vi "DSF.Execution.Runtime.Plugin Manager.Load Classes.vi"(8 "error in (no error)":errorcluster, 10 "class paths":path[](array[path]), 11 "Plugin Manager in":refnum<class "DSF.Engine.Runtime.Plugin Manager.lvclass">) -> (0 "error out":errorcluster, 2 "objects":refnum<class>[](array[class]), 3 "Plugin Manager out":refnum<class "DSF.Engine.Runtime.Plugin Manager.lvclass">)   [LabVIEW 2016, in "DSF.Engine.lvlib" / "DSF.Engine.Runtime.Plugin Manager.lvclass"]
uses:
  DSF.Engine.Runtime.Plugin Manager.lvclass
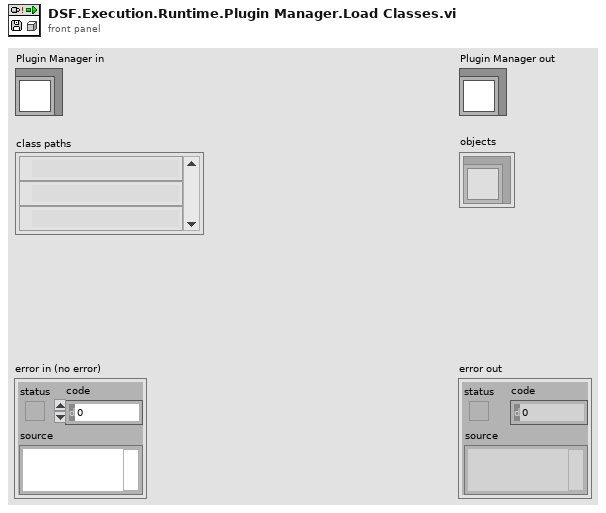
[diagram p1: front panel]
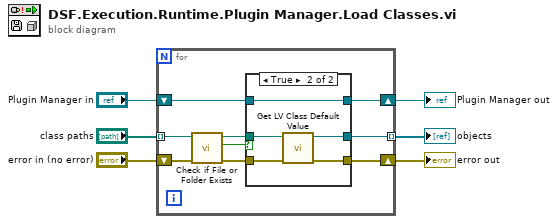
[diagram p0: block diagram]
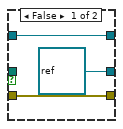
[diagram p2: hidden frame]
diagram:
  n1 = for {
    shift-right: [w10] -> w1
    shift-left: "error in (no error)" -> [w15]
    shift-right: [w7] -> w3
    shift-left: "Plugin Manager in" -> [w8]
    tunnel: "class paths" -> [w14] mode=indexing
    tunnel: [w9] -> w2 mode=indexing
    n2 = call <vilib>:"Check if File or Folder Exists.vi"("error in (no error)"=w15, "path"=w14) -> ("error out"=w12:errorcluster, "file or folder exists?"=w13:bool, "dup path"=w11:path)  [unwired: 7 in]
    n3 = case shown="True" w13 {
      tunnel: w12 -> [w17 w23]
      tunnel: w11 -> [_ w22]
      tunnel: [refnum<class> refnum ("object") w21] -> w9
      tunnel: [w17 w20] -> w10
      tunnel: w8 -> [w16 w19]
      tunnel: [w16 w19] -> w7
      frame False {
      }
      frame True {
        n4 = call <vilib>:"Get LV Class Default Value.vi"("error in (no error)"=w23, "class path"=w22) -> ("error out"=w20:errorcluster, "object"=w21:refnum<class>)  [unwired: 8 in]
      }
    }
  }
  "error out" <- w1
  "Plugin Manager out" <- w3
  "objects" <- w2
